vi "Create All Message Queues_Live.vi"(8 "error in (no error)":errorcluster) -> (0 "error out":errorcluster, 3 "Message Queues out":T1)   [LabVIEW 2019]
doc: "This VI creates and initializes all the message queues for your application. If your application requires more than one message queue, right-click the \"Message Queues\" constant above and select Open Type Def. Add the new Message Queue(s) to the type definition, then initialize them in this VI."
uses:
  All Message Queues.ctl
  Message Cluster.ctl
  Enqueue Message (Single).vi
  Message Queue.lvlib
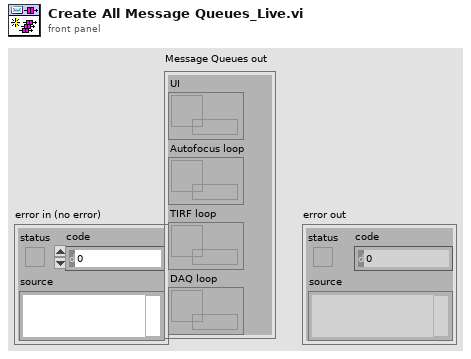
[diagram p1: front panel]
types:
  T1 = typedef "Message Queue.lvlib/All Message Queues.ctl" = cluster{"UI":refnum<queue>, "Autofocus loop":refnum<queue>, "TIRF loop":refnum<queue>, "DAQ loop":refnum<queue>}
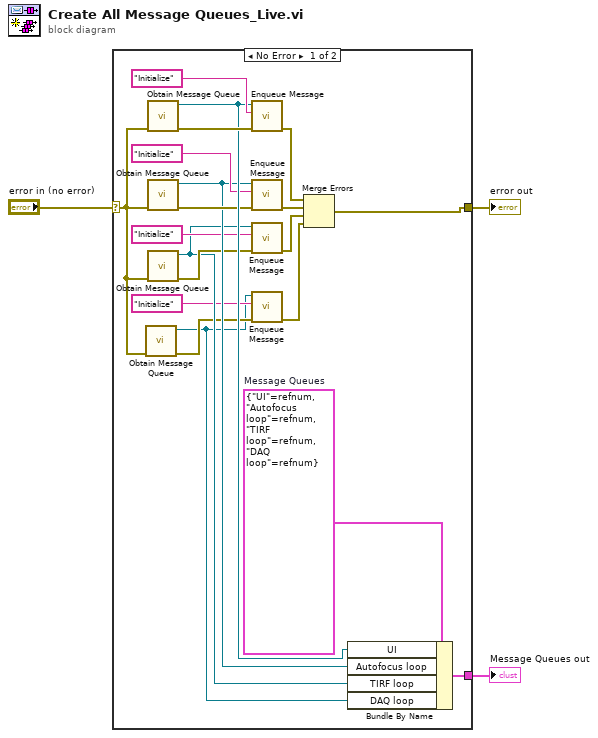
[diagram p0: block diagram]
diagram:
  n1 = case shown="No Error" "error in (no error)" {
    selector: "error in (no error)" -> [w6 w24]
    tunnel: [w14 w24] -> w3
    tunnel: [w22 _] -> w2
    frame No Error {
      w16 = T1 {"UI"=refnum, "Autofocus loop"=refnum, "TIRF loop"=refnum, "DAQ loop"=refnum}  # Message Queues
      n2 = call "Obtain Message Queue.vi"("error in (no error)"=w6) -> ("error out"=w8:errorcluster, "Message Queue"=w4:refnum<queue>)  [unwired: 9 in]
      n3 = call "Obtain Message Queue.vi"("error in (no error)"=w6) -> ("error out"=w21:errorcluster, "Message Queue"=w19:refnum<queue>)  [unwired: 9 in]
      n4 = call "Obtain Message Queue.vi"("error in (no error)"=w6) -> ("error out"=w18:errorcluster, "Message Queue"=w15:refnum<queue>)  [unwired: 9 in]
      n5 = call "Obtain Message Queue.vi"("error in (no error)"=w6) -> ("error out"=w12:errorcluster, "Message Queue"=w9:refnum<queue>)  [unwired: 9 in]
      n6 = call-poly "Enqueue Message.vi"("error in (no error)"=w21, "Message"="Initialize", "Message Queue"=w19) -> ("error out"=w23:errorcluster)  [unwired: 7 in, 1 out]
      n7 = call-poly "Enqueue Message.vi"("error in (no error)"=w18, "Message"="Initialize", "Message Queue"=w15) -> ("error out"=w13:errorcluster)  [unwired: 7 in, 1 out]
      n8 = call-poly "Enqueue Message.vi"("error in (no error)"=w12, "Message"="Initialize", "Message Queue"=w9) -> ("error out"=w10:errorcluster)  [unwired: 7 in, 1 out]
      n9 = call-poly "Enqueue Message.vi"("error in (no error)"=w8, "Message"="Initialize", "Message Queue"=w4) -> ("error out"=w5:errorcluster)  [unwired: 7 in, 1 out]
      n10 = Merge Errors(w23, w13, w10, w5) -> (w14:errorcluster)
      n11 = Bundle By Name(cluster=w16, "UI"=w19, "Autofocus loop"=w15, "TIRF loop"=w9, "DAQ loop"=w4) -> (w22:T1)
    }
    frame Error {
    }
  }
  "Message Queues out" <- w2
  "error out" <- w3
